vi "Refactored_GetLVDTParameters.vi"() -> ()   [LabVIEW 2016]
panel:
  out "Application":refnum<k7>
  out "error out":errorcluster
  in  "error in (no error)":errorcluster
  in  "Application":refnum<k7>
  out "YLVDT Offset":dbl
  out "XLVDT Offset":dbl
  out "YLVDT Sens":dbl
  out "XLVDT Sens":dbl
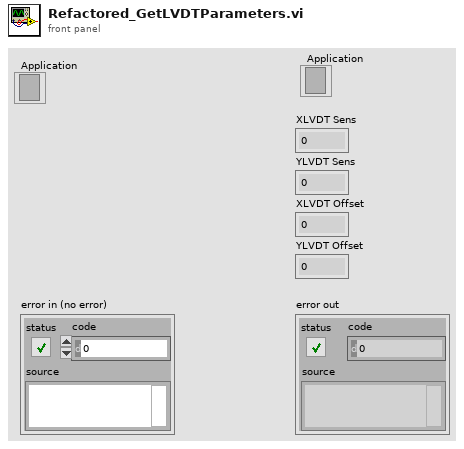
[diagram p1: front panel]
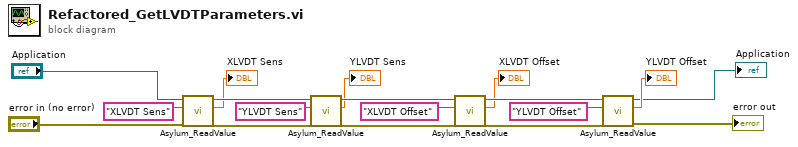
[diagram p0: block diagram]
diagram:
  n1 = call "Asylum_ReadValue.vi"("error in (no error)"="error in (no error)", "Value"="XLVDT Sens", "Application"="Application") -> ("error out"=w16:errorcluster, "Value"=→"XLVDT Sens":dbl, "Application"=w17:refnum<k7>)  [unwired: 6 in]
  n2 = call "Asylum_ReadValue.vi"("error in (no error)"=w16, "Value"="YLVDT Sens", "Application"=w17) -> ("error out"=w14:errorcluster, "Value"=→"YLVDT Sens":dbl, "Application"=w15:refnum<k7>)  [unwired: 6 in]
  n3 = call "Asylum_ReadValue.vi"("error in (no error)"=w14, "Value"="XLVDT Offset", "Application"=w15) -> ("error out"=w12:errorcluster, "Value"=→"XLVDT Offset":dbl, "Application"=w13:refnum<k7>)  [unwired: 6 in]
  n4 = call "Asylum_ReadValue.vi"("error in (no error)"=w12, "Value"="YLVDT Offset", "Application"=w13) -> ("error out"=→"error out":errorcluster, "Value"=→"YLVDT Offset":dbl, "Application"=→"Application":refnum<k7>)  [unwired: 6 in]
